vi "Rotation3d_Times.vi"(9 "Scalar":dbl, 11 "in Rotation3d":T1={"Q_quaternion"={"R"=1.0, "V"=[0.0, 0.0, 0.0]}}) -> (3 "out Rotation3d":T1={"Q_quaternion"={"R"=1.0, "V"=[0.0, 0.0, 0.0]}})   [LabVIEW 2019, in "Trajectory_Library.lvlib"]
doc: "Multiplies the current rotation (angle) by a scalar.\n\nParameters: \n- IN ROTATION - This ROTATION data structure\n- SCALAR - The value to multiiply the rotation by.\n\nReturns:\n - OUT ROTATION - THe new ROTATION data structure."
uses:
  Trajectory_Library.lvlib
  ROTATION3D.ctl
  QUATERNION.ctl
  Matrix_NormF.vi
  Quaternion_New.vi
  Rotation3d_Create_Default.vi
  <vilib>/Analysis/_algsub.llb/Matrix Norm.vi
  <vilib>/Analysis/_algsub.llb/Real Matrix Norm.vi
  Quaternion_New_Default.vi
  <vilib>/Analysis/Matrix/Numeric/Conversions/Array To Matrix.vi
  <vilib>/Analysis/Matrix/Numeric/Conversions/Array To Matrix - RA.vi
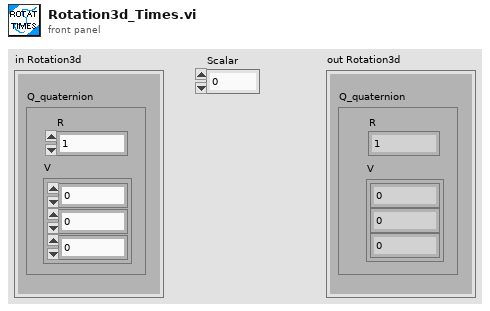
[diagram p1: front panel]
types:
  T1 = typedef "Trajectory_Library.lvlib/ROTATION3D.ctl" = cluster{"Q_quaternion":T2}
  T2 = typedef "Trajectory_Library.lvlib/QUATERNION.ctl" = cluster{"R":dbl, "V":dbl[]}
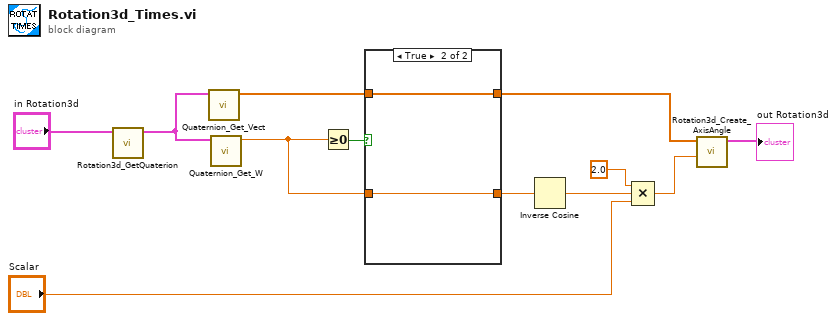
[diagram p0: block diagram]
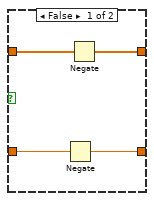
[diagram p2: hidden frame]
diagram:
  n1 = call "Rotation3d_GetQuaterion.vi"("in Rotation3d"="in Rotation3d") -> ("out Quaterion"=w1:T2)  [unwired: 10 in]
  n2 = call "Quaternion_Get_Vect.vi"("Quaternion"=w1) -> ("Vector"=w2:dbl[])  [unwired: 10 in]
  n3 = call "Quaternion_Get_W.vi"("Quaternion"=w1) -> ("W"=w8:dbl)  [unwired: 10 in]
  n4 = Greater Or Equal To 0?(x=w8) -> (x >= 0?=w12:bool)
  n5 = case shown="True" w12 {
    tunnel: w2 -> [w13 w18]
    tunnel: [w14 w18] -> w10
    tunnel: w8 -> [w16 w17]
    tunnel: [w15 w17] -> w7
    frame False {
      n6 = Negate(x=w16) -> (-x=w15:dbl)
      n7 = Negate(x=w13) -> (-x=w14:dbl[])
    }
    frame True {
    }
  }
  n8 = Inverse Cosine(1:w7) -> (0:w6:dbl)
  n9 = Compound Arithmetic op=MULTIPLY(2.0 ("value"), w6, "Scalar") -> (w5:dbl)
  n10 = call "Rotation3d_Create_AxisAngle.vi"("Angle"=w5, "Axis Vector"=w10) -> ("Rotation3d"=→"out Rotation3d":T1)  [unwired: 9 in]
